vi "ABB Size 2D array.vi"(5 "Type":enum16{"Integer", "DBL", "STRING", "BOOLEAN"}(ring), 6 "Defaults":T1 {"Dbl" format="%.2f"}, 7 "Size":cluster{"# rows":i32, "# cols":i32}, 8 "Boolean Array in":bool[][](array[boolean]), 9 "String Array in":string[][](array[string]), 10 "DBL Array In":dbl[][](array[numeric]) format="%.2f", 11 "Integer Array In":i32[][](array[numeric])) -> (0 "Boolean Array out":bool[][](array[boolean]), 1 "String Array out":string[][](array[string]), 2 "DBL Array out":dbl[][](array[numeric]) format="%.2f", 3 "Integer Array Out":i32[][](array[numeric]))   [LabVIEW 2017]
panel:
  in  "Default type":enum16{"All", "Row", "Column"}(ring)
  out "O/P size":i32[](array[numeric])
  out "Dcol":i32
  out "Drow":i32
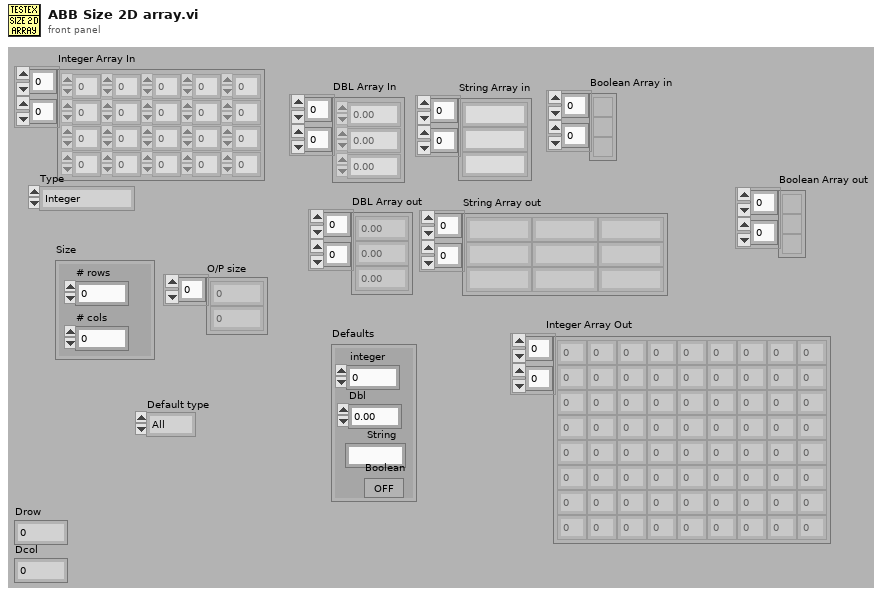
[diagram p1: front panel]
types:
  T1 = cluster{" integer":i32, "Dbl":dbl, " String":string, "Boolean":bool}
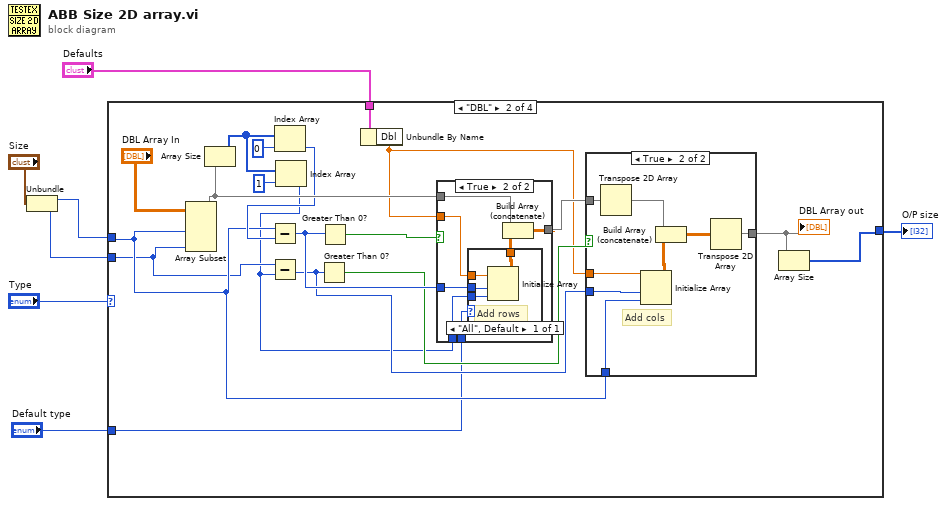
[diagram p0: block diagram]
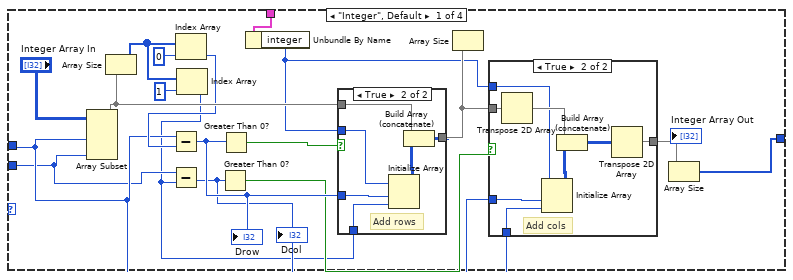
[diagram p2: hidden frame]
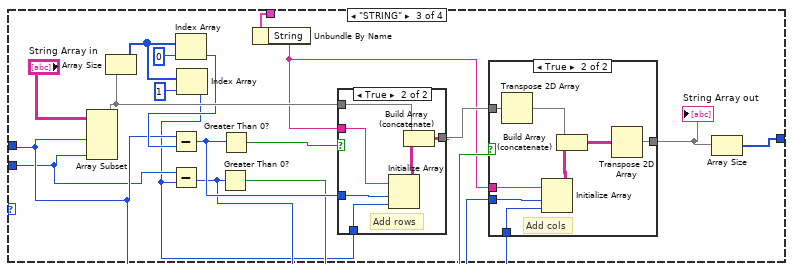
[diagram p7: hidden frame]
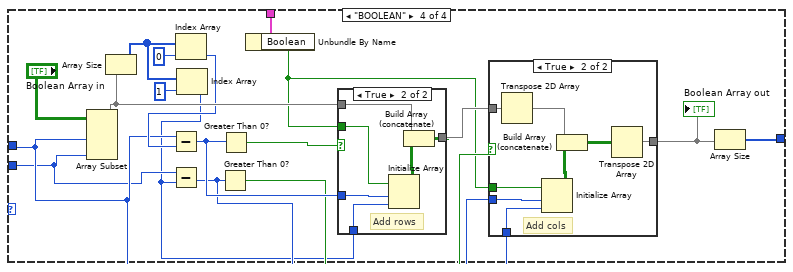
[diagram p10: hidden frame]
diagram:
  n1 = Unbundle("Size") -> ("# rows"=w5:i32, "# cols"=w4:i32)
  n2 = case shown="\"DBL\"" "Type" {
    tunnel: w5 -> [w16 w52 w91 w125]
    tunnel: w4 -> [w13 w50 w89 w123]
    tunnel: [w10 w45 w84 w118] -> w3
    tunnel: "Defaults" -> [w9 w44 w83 w117]
    tunnel: "Default type" -> [_ w42 _ _]
    frame "Integer", Default {
      n3 = Array Subset(array="Integer Array In", length (row)=w16, length (col)=w13) -> (w24:i32[][])  [unwired: 2 in]
      n4 = Array Size(array=w24) -> (size(s)=w20:i32[])
      n5 = Index Array(array=w20, index=0 ("Index")) -> (element=w22:i32)
      n6 = Subtract(x=w16, y=w22) -> (x-y=w18:i32)
      "Drow" <- w18
      n7 = Index Array(array=w20, index=1 ("Index")) -> (element=w12:i32)
      n8 = Subtract(x=w13, y=w12) -> (x-y=w17:i32)
      "Dcol" <- w17
      n9 = Greater Than 0?(x=w17) -> (x > 0?=w15:bool)
      n10 = Greater Than 0?(x=w18) -> (x > 0?=w19:bool)
      n11 = Unbundle By Name(w9) -> ("integer"=w8:i32)
      n12 = case shown="True" w19 {
        tunnel: w18 -> [_ w41]
        tunnel: w24 -> [w35 w40]
        tunnel: [w35 w38] -> w14
        tunnel: w12 -> [_ w37]
        tunnel: w8 -> [_ w36]
        frame False {
        }
        frame True {
          # "Add rows"
          n13 = Initialize Array(w36, w41, w37) -> (w39:i32[][])
          n14 = Build Array (concatenate)(w40, w39) -> (w38:i32[][])
        }
      }
      n15 = Array Size(array=w14) -> ()  [unwired: 1 out]
      n16 = case shown="True" w15 {
        tunnel: w17 -> [_ w34]
        tunnel: w14 -> [w26 w33]
        tunnel: [w26 w28] -> w11
        tunnel: w16 -> [_ w30]
        tunnel: w8 -> [_ w27]
        frame False {
        }
        frame True {
          # "Add cols"
          n17 = Transpose 2D Array(2D array=w33) -> (transposed array=w29:i32[][])
          n18 = Initialize Array(w27, w34, w30) -> (w32:i32[][])
          n19 = Build Array (concatenate)(w29, w32) -> (w31:i32[][])
          n20 = Transpose 2D Array(2D array=w31) -> (transposed array=w28:i32[][])
        }
      }
      "Integer Array Out" <- w11
      n21 = Array Size(array=w11) -> (size(s)=w10:i32[])
    }
    frame "DBL" {
      n22 = Array Subset(array="DBL Array In", length (row)=w52, length (col)=w50) -> (w60:dbl[][])  [unwired: 2 in]
      n23 = Array Size(array=w60) -> (size(s)=w56:i32[])
      n24 = Index Array(array=w56, index=0 ("Index")) -> (element=w58:i32)
      n25 = Subtract(x=w52, y=w58) -> (x-y=w54:i32)
      n26 = Index Array(array=w56, index=1 ("Index")) -> (element=w49:i32)
      n27 = Subtract(x=w50, y=w49) -> (x-y=w53:i32)
      n28 = Greater Than 0?(x=w53) -> (x > 0?=w51:bool)
      n29 = Greater Than 0?(x=w54) -> (x > 0?=w55:bool)
      n30 = Unbundle By Name(w44) -> ("Dbl"=w43:dbl)
      n31 = case shown="True" w55 {
        tunnel: w54 -> [_ w77]
        tunnel: w60 -> [w70 w76]
        tunnel: [w70 w74] -> w47
        tunnel: w49 -> [_ w73]
        tunnel: w43 -> [_ w72]
        tunnel: w42 -> [_ w71]
        frame False {
        }
        frame True {
          n32 = case shown="\"All\", Default" w71 {
            tunnel: w77 -> [w81]
            tunnel: [w80] -> w75
            tunnel: w73 -> [w79]
            tunnel: w72 -> [w78]
            frame "All", Default {
              # "Add rows"
              n33 = Initialize Array(w78, w81, w79) -> (w80:dbl[][])
            }
          }
          n34 = Build Array (concatenate)(w76, w75) -> (w74:dbl[][])
        }
      }
      n35 = case shown="True" w51 {
        tunnel: w53 -> [_ w69]
        tunnel: w47 -> [w61 w68]
        tunnel: [w61 w63] -> w46
        tunnel: w52 -> [_ w65]
        tunnel: w43 -> [_ w62]
        frame False {
        }
        frame True {
          # "Add cols"
          n36 = Transpose 2D Array(2D array=w68) -> (transposed array=w64:dbl[][])
          n37 = Initialize Array(w62, w69, w65) -> (w67:dbl[][])
          n38 = Build Array (concatenate)(w64, w67) -> (w66:dbl[][])
          n39 = Transpose 2D Array(2D array=w66) -> (transposed array=w63:dbl[][])
        }
      }
      "DBL Array out" <- w46
      n40 = Array Size(array=w46) -> (size(s)=w45:i32[])
    }
    frame "STRING" {
      n41 = Array Subset(array="String Array in", length (row)=w91, length (col)=w89) -> (w99:string[][])  [unwired: 2 in]
      n42 = Array Size(array=w99) -> (size(s)=w95:i32[])
      n43 = Index Array(array=w95, index=0 ("Index")) -> (element=w97:i32)
      n44 = Subtract(x=w91, y=w97) -> (x-y=w93:i32)
      n45 = Index Array(array=w95, index=1 ("Index")) -> (element=w88:i32)
      n46 = Subtract(x=w89, y=w88) -> (x-y=w92:i32)
      n47 = Greater Than 0?(x=w92) -> (x > 0?=w90:bool)
      n48 = Greater Than 0?(x=w93) -> (x > 0?=w94:bool)
      n49 = Unbundle By Name(w83) -> ("String"=w82:string)
      n50 = case shown="True" w94 {
        tunnel: w93 -> [_ w115]
        tunnel: w99 -> [w109 w114]
        tunnel: [w109 w112] -> w87
        tunnel: w88 -> [_ w111]
        tunnel: w82 -> [_ w110]
        frame False {
        }
        frame True {
          # "Add rows"
          n51 = Initialize Array(w110, w115, w111) -> (w113:string[][])
          n52 = Build Array (concatenate)(w114, w113) -> (w112:string[][])
        }
      }
      n53 = case shown="True" w90 {
        tunnel: w92 -> [_ w108]
        tunnel: w87 -> [w100 w107]
        tunnel: [w100 w102] -> w85
        tunnel: w91 -> [_ w104]
        tunnel: w82 -> [_ w101]
        frame False {
        }
        frame True {
          # "Add cols"
          n54 = Transpose 2D Array(2D array=w107) -> (transposed array=w103:string[][])
          n55 = Initialize Array(w101, w108, w104) -> (w106:string[][])
          n56 = Build Array (concatenate)(w103, w106) -> (w105:string[][])
          n57 = Transpose 2D Array(2D array=w105) -> (transposed array=w102:string[][])
        }
      }
      "String Array out" <- w85
      n58 = Array Size(array=w85) -> (size(s)=w84:i32[])
    }
    frame "BOOLEAN" {
      n59 = Array Subset(array="Boolean Array in", length (row)=w125, length (col)=w123) -> (w133:bool[][])  [unwired: 2 in]
      n60 = Array Size(array=w133) -> (size(s)=w129:i32[])
      n61 = Index Array(array=w129, index=0 ("Index")) -> (element=w131:i32)
      n62 = Subtract(x=w125, y=w131) -> (x-y=w127:i32)
      n63 = Index Array(array=w129, index=1 ("Index")) -> (element=w122:i32)
      n64 = Subtract(x=w123, y=w122) -> (x-y=w126:i32)
      n65 = Greater Than 0?(x=w126) -> (x > 0?=w124:bool)
      n66 = Greater Than 0?(x=w127) -> (x > 0?=w128:bool)
      n67 = Unbundle By Name(w117) -> ("Boolean"=w116:bool)
      n68 = case shown="True" w128 {
        tunnel: w127 -> [_ w149]
        tunnel: w133 -> [w143 w148]
        tunnel: [w143 w146] -> w121
        tunnel: w122 -> [_ w145]
        tunnel: w116 -> [_ w144]
        frame False {
        }
        frame True {
          # "Add rows"
          n69 = Initialize Array(w144, w149, w145) -> (w147:bool[][])
          n70 = Build Array (concatenate)(w148, w147) -> (w146:bool[][])
        }
      }
      n71 = case shown="True" w124 {
        tunnel: w126 -> [_ w142]
        tunnel: w121 -> [w134 w141]
        tunnel: [w134 w136] -> w119
        tunnel: w125 -> [_ w138]
        tunnel: w116 -> [_ w135]
        frame False {
        }
        frame True {
          # "Add cols"
          n72 = Transpose 2D Array(2D array=w141) -> (transposed array=w137:bool[][])
          n73 = Initialize Array(w135, w142, w138) -> (w140:bool[][])
          n74 = Build Array (concatenate)(w137, w140) -> (w139:bool[][])
          n75 = Transpose 2D Array(2D array=w139) -> (transposed array=w136:bool[][])
        }
      }
      "Boolean Array out" <- w119
      n76 = Array Size(array=w119) -> (size(s)=w118:i32[])
    }
  }
  "O/P size" <- w3
